vi "Close.vi"(8 "error in (no error)":errorcluster, 11 "AO Ref In":T1) -> (0 "error out":errorcluster)   [LabVIEW 2021, in "AO.lvlib"]
doc: "Closes the reference to one or more analog output channels and resets the output voltage to 0 V."
uses:
  <vilib>/myRIO/Instrument Drivers/Onboard IO/AO/AO.lvlib
  <vilib>/myRIO/Instrument Drivers/Onboard IO/AO/typedefs/AO Reference.ctl
  <vilib>/myRIO/Common/Instrument Driver Framework/Utilities/typedefs/myRIO Generic Hardware Reference.ctl
  <vilib>/myRIO/Common/Instrument Driver Framework/Utilities/typedefs/Hardware Version Enum.ctl
  <vilib>/myRIO/Common/Instrument Driver Framework/Utilities/typedefs/myRIO v1.0 Reference.ctl
  <vilib>/myRIO/Common/Instrument Driver Framework/Utilities/typedefs/Generic FPGA Reference.ctl
  <vilib>/myRIO/Common/Instrument Driver Framework/myRIO v1.0/AO/typedefs/AO Channels List.ctl
  <vilib>/myRIO/Common/Instrument Driver Framework/myRIO v1.0/AO/typedefs/AO Channels Enum.ctl
  <vilib>/myRIO/Common/Instrument Driver Framework/Utilities/typedefs/Analog Scaling Constants List.ctl
  <vilib>/myRIO/Common/Instrument Driver Framework/Utilities/typedefs/Analog Scaling Constants.ctl
  <vilib>/myRIO/Common/Instrument Driver Framework/myRIO v1.0/AO/vis/myRIO v1.0 Unreserve AO.vi
  <vilib>/myRIO/Common/Instrument Driver Framework/roboRIO v1.0/AO/vis/roboRIO v1.0 Unreserve AO.vi
  <vilib>/myRIO/Common/Instrument Driver Framework/ELVIS III v1.0/AO/vis/ELVIS III v1.0 Unreserve AO.vi
  <vilib>/myRIO/Common/Instrument Driver Framework/myRIO v1.0/Resource Manager/vis/myRIO v1.0 Unreserve Channel List.vi
  <vilib>/myRIO/Common/Instrument Driver Framework/myRIO v1.0/AO/vis/myRIO v1.0 Build MUX Configuration AO.vi
  <vilib>/myRIO/Common/Instrument Driver Framework/roboRIO v1.0/AO/vis/roboRIO v1.0 Build MUX Configuration AO.vi
  <vilib>/myRIO/Common/Instrument Driver Framework/roboRIO v1.0/Resource Manager/vis/roboRIO v1.0 Unreserve Channel List.vi
  <vilib>/myRIO/Common/Instrument Driver Framework/ELVIS III v1.0/AO/vis/ELVIS III v1.0 Build MUX Configuration AO.vi
  <vilib>/myRIO/Common/Instrument Driver Framework/myRIO v1.0/Resource Manager/vis/myRIO v1.0 Unreserve Channel.vi
  <vilib>/myRIO/Common/Instrument Driver Framework/roboRIO v1.0/Resource Manager/vis/roboRIO v1.0 Unreserve Channel.vi
  <vilib>/myRIO/Common/Instrument Driver Framework/myRIO v1.0/Resource Manager/vis/myRIO v1.0 Build Mutex Name.vi
  <vilib>/myRIO/Common/Instrument Driver Framework/roboRIO v1.0/Resource Manager/vis/roboRIO v1.0 Build Mutex Name.vi
  <vilib>/myRIO/Common/Instrument Driver Framework/myRIO v1.0/AO/vis/myRIO v1.0 Write AO.vi
  <vilib>/myRIO/Common/Instrument Driver Framework/Utilities/vis/Configuration Manager.vi
  <vilib>/myRIO/Common/Instrument Driver Framework/Utilities/vis/IO Manager.vi
  <vilib>/myRIO/Common/Instrument Driver Framework/roboRIO v1.0/AO/vis/roboRIO v1.0 Write AO.vi
  <vilib>/myRIO/Common/Instrument Driver Framework/ELVIS III v1.0/AO/vis/ELVIS III v1.0 Write AO.vi
  <vilib>/myRIO/Common/Instrument Driver Framework/ELVIS III v1.0/Resource Manager/vis/ELVIS III v1.0 Unreserve Channel List.vi
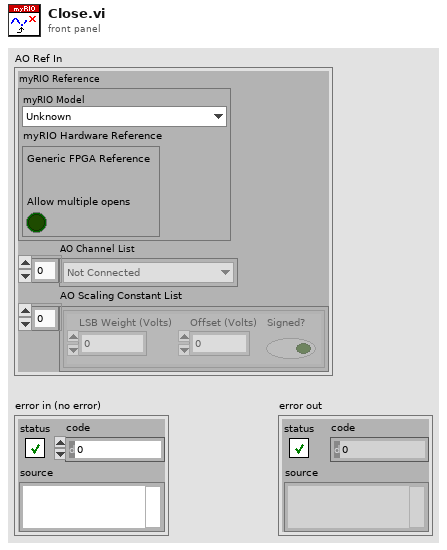
[diagram p1: front panel]
types:
  T1 = typedef "AO.lvlib/AO Reference.ctl" = cluster{"myRIO Reference":T2, "AO Channel List":T6, "AO Scaling Constant List":T8}
  T2 = typedef "myRIO Generic Hardware Reference.ctl" = cluster{"myRIO Model":T3, "myRIO Hardware Reference":T4}
  T3 = typedef "Hardware Version Enum.ctl" = enum16{"Unknown", "myRIO-1900", "myRIO-1950", "roboRIO", "NI ELVIS RIO CM", "ELVIS III"}
  T4 = typedef "myRIO v1.0 Reference.ctl" = cluster{"Generic FPGA Reference":T5, "Allow multiple opens":bool}
  T5 = typedef "Generic FPGA Reference.ctl" = refnum<k20>
  T6 = typedef "AO Channels List.ctl" = T7[]
  T7 = typedef "AO Channels Enum.ctl" = enum16{"Not Connected", "AudioOut/Left", "AudioOut/Right", "C/AO0", "C/AO1", "A/AO0", "A/AO1", "B/AO0", "B/AO1"}
  T8 = typedef "Analog Scaling Constants List.ctl" = T9[]
  T9 = typedef "Analog Scaling Constants.ctl" = cluster{"LSB Weight (Volts)":dbl, "Offset (Volts)":dbl, "Signed?":bool}
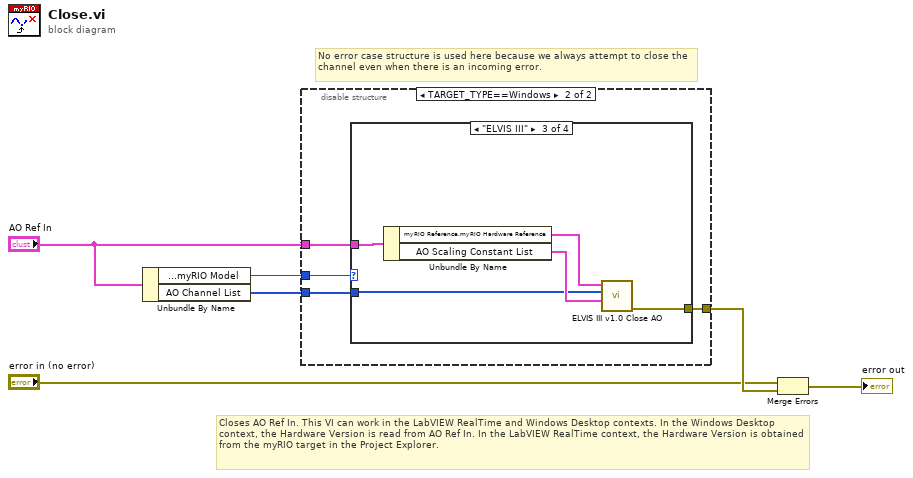
[diagram p0: block diagram]
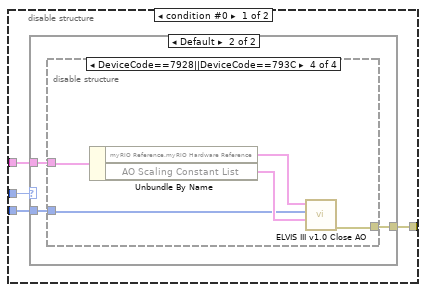
[diagram p2: hidden frame]
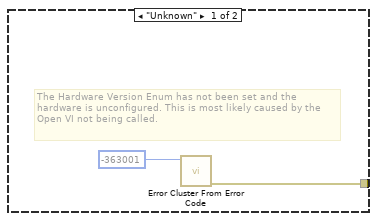
[diagram p3: hidden frame]
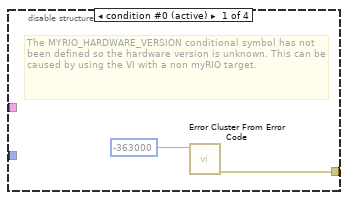
[diagram p4: hidden frame]
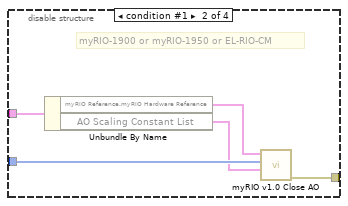
[diagram p5: hidden frame]
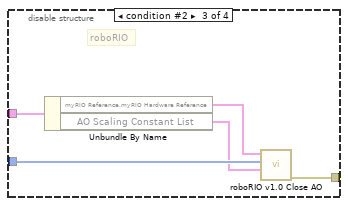
[diagram p6: hidden frame]
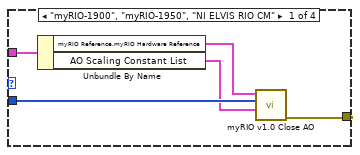
[diagram p7: hidden frame]
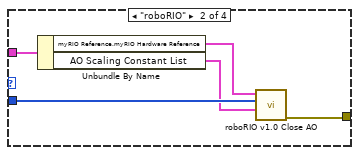
[diagram p8: hidden frame]
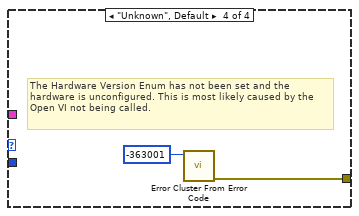
[diagram p9: hidden frame]
diagram:
  # "No error case structure is used here because we always attempt to close the channel even when there is an incoming error."
  # "Closes AO Ref In. This VI can work in the LabVIEW RealTime and Windows Desktop contexts. In the Windows Desktop context, the Hardware Version is read from AO Ref In. In the LabVIEW RealTime context, the Hardware Version is obtained from the myRIO target in the Project Explorer."
  n1 = Unbundle By Name("AO Ref In") -> ("myRIO Reference.myRIO Model"=w2:T3, "AO Channel List"=w1:T6)
  n2 = disable-structure shown="TARGET_TYPE==Windows" {
    disable-tunnel: "AO Ref In" -> [w10 w35]
    disable-tunnel: [w9 w36] -> w6
    disable-tunnel: w2 -> [w8 w34]
    disable-tunnel: w1 -> [w7 w33]
    frame condition #0 {
      n3 = case shown="Default" w8 {
        tunnel: w10 -> [_ w15]
        tunnel: [w11 w14] -> w9
        tunnel: w7 -> [_ w13]
        frame "Unknown" {
          # "The Hardware Version Enum has not been set and the hardware is unconfigured. This is most likely caused by the Open VI not being called."
          n4 = call <vilib>:"Error Cluster From Error Code.vi"("error code (0)"=-363001) -> ("error out"=w11:errorcluster)  [unwired: 8 in]
        }
        frame Default {
          n5 = disable-structure shown="DeviceCode==7928||DeviceCode==793C" {
            disable-tunnel: w15 -> [_ w22 w27 w30]
            disable-tunnel: [w16 w21 w26 w28] -> w14
            disable-tunnel: w13 -> [_ w20 w25 w29]
            frame condition #0 (active) {
              # "The MYRIO_HARDWARE_VERSION conditional symbol has not been defined so the hardware version is unknown. This can be caused by using the VI with a non myRIO target."
              n6 = call <vilib>:"Error Cluster From Error Code.vi"("error code (0)"=-363000) -> ("error out"=w16:errorcluster)  [unwired: 8 in]
            }
            frame condition #1 {
              # "myRIO-1900 or myRIO-1950 or EL-RIO-CM"
              n7 = Unbundle By Name(w22) -> ("myRIO Reference.myRIO Hardware Reference"=w19:T4, "AO Scaling Constant List"=w18:T8)
              n8 = call <vilib>:"myRIO v1.0 Close AO.vi"("Scale Constants Array"=w18, "AO Channel List"=w20, "myRIO Ref In"=w19) -> ("error out"=w21:errorcluster)  [unwired: 8 in]
            }
            frame condition #2 {
              # "roboRIO"
              n9 = Unbundle By Name(w27) -> ("myRIO Reference.myRIO Hardware Reference"=w24:T4, "AO Scaling Constant List"=w23:T8)
              n10 = call <vilib>:"roboRIO v1.0 Close AO.vi"("Scale Constants Array"=w23, "AO Channel List"=w25, "myRIO Ref In"=w24) -> ("error out"=w26:errorcluster)  [unwired: 8 in]
            }
            frame condition #3 {
              n11 = Unbundle By Name(w30) -> ("myRIO Reference.myRIO Hardware Reference"=w32:T4, "AO Scaling Constant List"=w31:T8)
              n12 = call <vilib>:"ELVIS III v1.0 Close AO.vi"("Scale Constants Array"=w31, "AO Channel List"=w29, "myRIO Ref In"=w32) -> ("error out"=w28:errorcluster)  [unwired: 8 in]
            }
          }
        }
      }
    }
    frame condition #1 (active) {
      n13 = case shown="\"ELVIS III\"" w34 {
        tunnel: w35 -> [w41 w46 w47 _]
        tunnel: [w40 w45 w49 w52] -> w36
        tunnel: w33 -> [w38 w43 w48 _]
        frame "myRIO-1900", "myRIO-1950", "NI ELVIS RIO CM" {
          n14 = Unbundle By Name(w41) -> ("myRIO Reference.myRIO Hardware Reference"=w39:T4, "AO Scaling Constant List"=w37:T8)
          n15 = call <vilib>:"myRIO v1.0 Close AO.vi"("Scale Constants Array"=w37, "AO Channel List"=w38, "myRIO Ref In"=w39) -> ("error out"=w40:errorcluster)  [unwired: 8 in]
        }
        frame "roboRIO" {
          n16 = Unbundle By Name(w46) -> ("myRIO Reference.myRIO Hardware Reference"=w44:T4, "AO Scaling Constant List"=w42:T8)
          n17 = call <vilib>:"roboRIO v1.0 Close AO.vi"("Scale Constants Array"=w42, "AO Channel List"=w43, "myRIO Ref In"=w44) -> ("error out"=w45:errorcluster)  [unwired: 8 in]
        }
        frame "ELVIS III" {
          n18 = Unbundle By Name(w47) -> ("myRIO Reference.myRIO Hardware Reference"=w51:T4, "AO Scaling Constant List"=w50:T8)
          n19 = call <vilib>:"ELVIS III v1.0 Close AO.vi"("Scale Constants Array"=w50, "AO Channel List"=w48, "myRIO Ref In"=w51) -> ("error out"=w49:errorcluster)  [unwired: 8 in]
        }
        frame "Unknown", Default {
          # "The Hardware Version Enum has not been set and the hardware is unconfigured. This is most likely caused by the Open VI not being called."
          n20 = call <vilib>:"Error Cluster From Error Code.vi"("error code (0)"=-363001) -> ("error out"=w52:errorcluster)  [unwired: 8 in]
        }
      }
    }
  }
  n21 = Merge Errors("error in (no error)", w6) -> (→"error out":errorcluster)
